vi "Get configuration chain.vi"(8 "error in (no error)":errorcluster, 11 "ThorcamBase in":refnum<class "Thorcam.lvclass">) -> (0 "error out":errorcluster, 1 "class name":string[](array[string]), 2 "configuration chain":variant[](array[variant]), 3 "ThorcamBase out":refnum<class "Thorcam.lvclass">)   [LabVIEW 2012, in "Thorcam.lvclass"]
doc: "Returns an array of variants containing the configuration clusters of each class in the inheritance chain (lowest child class first), together with an array of all class names in the inheritance chain.\n\nFor classes without configuration cluster, the configuration chain contains empty variants."
uses:
  Thorcam.lvclass
  <vilib>/Distrio/Murmex/Murmex/Murmex.lvclass
  Thorcam.lvclass/Thorcam.ctl
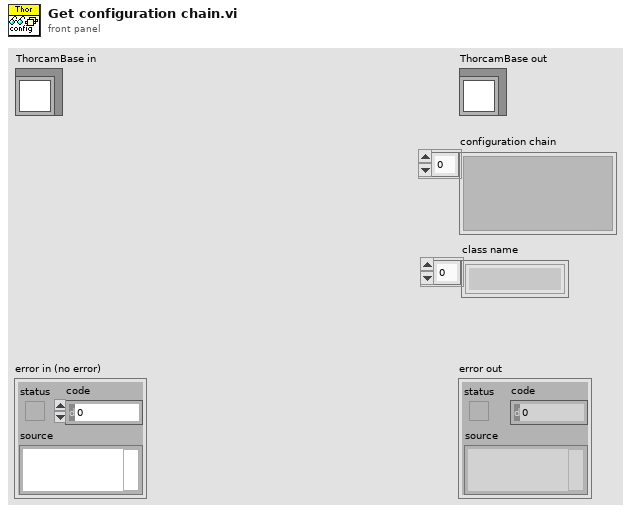
[diagram p1: front panel]
types:
  T1 = typedef "Thorcam.lvclass/configuration.ctl" = cluster{"camera ID1":u32, "Settings":string, "Cross Correlation method":T2, "Reporting folder":path, "LUT":path, "Stage component":string, "Background image":path, "camera ID2":u32, "select camera":u32, "Shift to defocus conversion factor":dbl, "Alignment quality threshold":dbl, "shutter control digital line":string}
  T2 = typedef "Thorcam.lvclass/cross correlation method.ctl" = enum16{"default", "normalised cross correlation", "normalised mutual information", "binary cross correlation", "binary mutual information"}
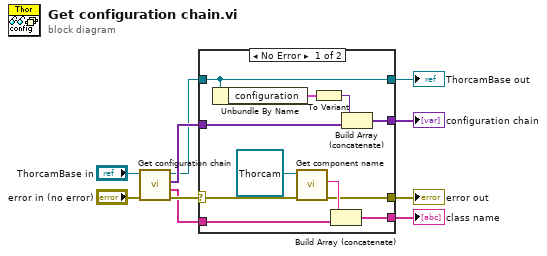
[diagram p0: block diagram]
diagram:
  n1 = call-parent "Get configuration chain.vi"("error in (no error)"="error in (no error)", "MurmexBase in"="ThorcamBase in") -> ("error out"=w8:errorcluster, "class name"=w6:string[], "configuration chain"=w4:variant[], "MurmexBase out"=w2:refnum<class "Thorcam.lvclass">)  [unwired: 6 in]
  n2 = case shown="No Error" w8 {
    selector: w8 -> [w19 w22]
    tunnel: [w18 w22] -> w7
    tunnel: w6 -> [w16 _]
    tunnel: [w15 _] -> w5
    tunnel: w4 -> [w14 _]
    tunnel: [w13 _] -> w3
    tunnel: w2 -> [w12 w23]
    tunnel: [w12 w23] -> w1
    frame No Error {
      n3 = Unbundle By Name(w12) -> ("configuration"=w11:T1)
      n4 = call <vilib>:"Get component name.vi"("error in (no error)"=w19, "Murmex in"=refnum<class "Thorcam.lvclass"> refnum ("Thorcam")) -> ("error out"=w18:errorcluster, "component name"=w21:string)  [unwired: 7 in, 1 out]
      n5 = To Variant(anything=w11) -> (Variant=w20:variant)
      n6 = Build Array (concatenate)(w21, w16) -> (w15:string[])
      n7 = Build Array (concatenate)(w20, w14) -> (w13:variant[])
    }
    frame Error {
    }
  }
  "error out" <- w7
  "ThorcamBase out" <- w1
  "configuration chain" <- w3
  "class name" <- w5
